vi "read button list.vi"(8 "Error In":errorcluster, 11 "ButtonList":refnum<k24>[](array[refnum])) -> (0 "Error Out":errorcluster, 2 "Button List":T1[](array[typedef]))   [LabVIEW 2015, in "Configuration Tool.lvlib"]
uses:
  Configuration Tool.lvlib
  XML Controls/Button.ctl
  XML Controls/Path Cluster.ctl
  XML Controls/Button Type.ctl
  XML Controls/Dependency three item small.ctl
  NationalInstruments.VeriStand.XMLReader
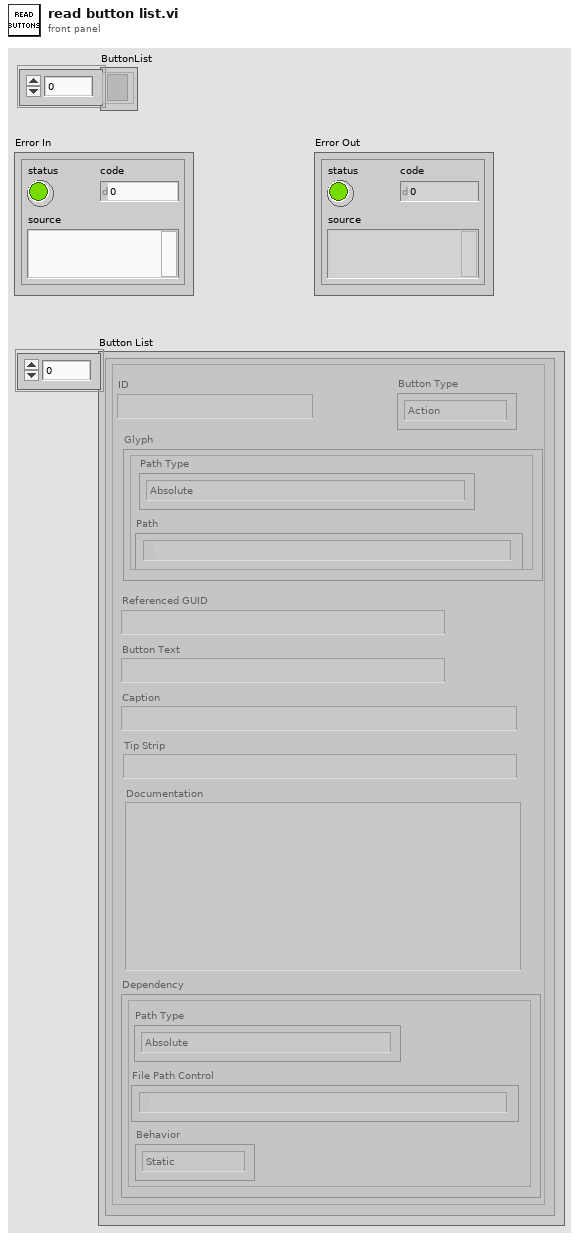
[diagram p1: front panel]
types:
  T1 = typedef "Configuration Tool.lvlib/Button.ctl" = cluster{"ID":string, "Glyph":T2, "Button Type":T3, "Referenced GUID":string, "Button Text":string, "Caption":string, "Tip Strip":string, "Documentation":string, "Dependency":T4}
  T2 = typedef "Configuration Tool.lvlib/Path Cluster.ctl" = cluster{"Path":path, "Path Type":enum16{"Absolute", "To Base", "To Common Doc Dir", "To Application Data Dir"}}
  T3 = typedef "Configuration Tool.lvlib/Button Type.ctl" = enum16{"Action", "Dialog", "Page", "Notification", "Separator"}
  T4 = typedef "Configuration Tool.lvlib/Dependency three item small.ctl" = cluster{"File Path Control":path, "Path Type":enum16{"Absolute", "To Base", "To Common Doc Dir", "To Application Data Dir"}, "Behavior":enum16{"Static", "Dynamic"}}
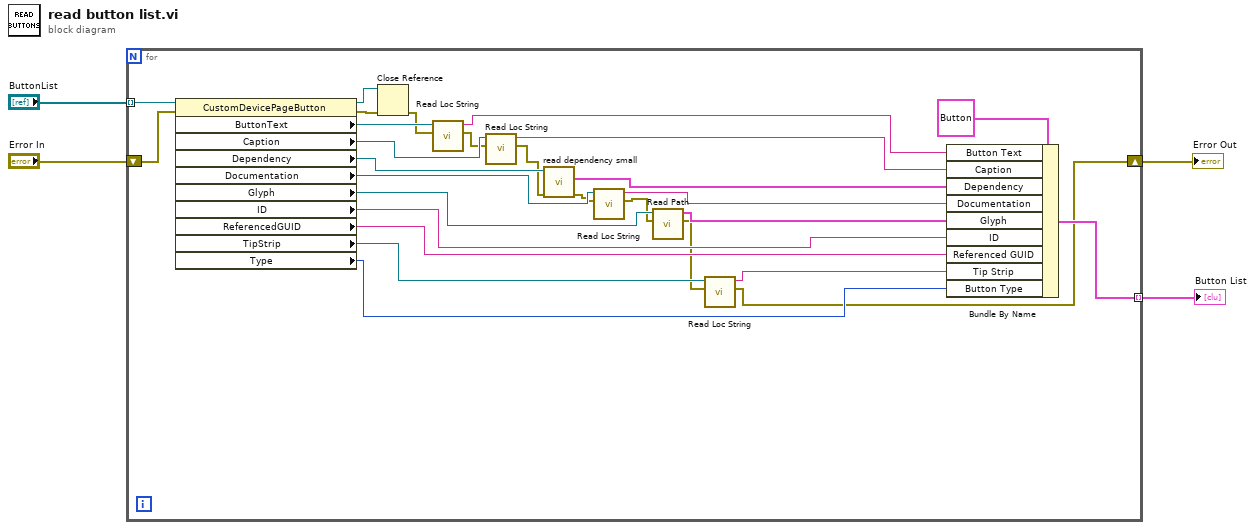
[diagram p0: block diagram]
diagram:
  n1 = for {
    tunnel: "ButtonList" -> [w32] mode=indexing
    shift-right: [w7] -> w2
    shift-left: "Error In" -> [w29]
    tunnel: [w27] -> w1 mode=indexing
    n2 = property class="CustomDevicePageButton"(reference=w32, error in=w29) -> (reference out=w31:refnum<k24>, error out=w30:errorcluster, "ButtonText"=w26:refnum<k24>, "Caption"=w25:refnum<k24>, "Dependency"=w24:refnum<k24>, "Documentation"=w23:refnum<k24>, "Glyph"=w22:refnum<k24>, "ID"=w21:string, "ReferencedGUID"=w20:string, "TipStrip"=w19:refnum<k24>, "Type"=w18:i32)
    n3 = Close Reference(reference=w31, error in (no error)=w30) -> (error out=w16:errorcluster)
    n4 = call "Read Loc String.vi"("Error In"=w16, "Loc String .NET Ref"=w26) -> ("Error Out"=w13:errorcluster, "English"=w15:string)  [unwired: 7 in, 1 out]
    n5 = call "Read Loc String.vi"("Error In"=w13, "Loc String .NET Ref"=w25) -> ("Error Out"=w12:errorcluster, "English"=w14:string)  [unwired: 7 in, 1 out]
    n6 = call "read dependency small.vi"("error in (no error)"=w12, ".NET Refnum in"=w24) -> ("error out"=w11:errorcluster, "Dependency"=w17:T4)  [unwired: 8 in]
    n7 = call "Read Loc String.vi"("Error In"=w11, "Loc String .NET Ref"=w23) -> ("Error Out"=w10:errorcluster, "English"=w5:string)  [unwired: 7 in, 1 out]
    n8 = call "Read Path.vi"("Error In"=w10, "Path .NET Ref"=w22) -> ("Error Out"=w8:errorcluster, "Path Properties"=w9:T2)  [unwired: 8 in]
    n9 = call "Read Loc String.vi"("Error In"=w8, "Loc String .NET Ref"=w19) -> ("Error Out"=w7:errorcluster, "English"=w6:string)  [unwired: 7 in, 1 out]
    n10 = Bundle By Name(cluster=T1 {"ID"="", "Glyph"={"Path"=path "", "Path Type"=enum."Absolute"}, "Button Type"=enum."Action", "Referenced GUID"="", "Button Text"="", "Caption"="", "Tip Strip"="", "Documentation"="", "Dependency"={"File Path Control"=path "", "Path Type"=enum."Absolute", "Behavior"=enum."Static"}} ("Button"), "Button Text"=w15, "Caption"=w14, "Dependency"=w17, "Documentation"=w5, "Glyph"=w9, "ID"=w21, "Referenced GUID"=w20, "Tip Strip"=w6, "Button Type"=w18) -> (w27:T1)
  }
  "Button List" <- w1
  "Error Out" <- w2
